vi "SLMLabv1 Test.vi"() -> ()   [LabVIEW 2019]
uses:
  <vilib>/vision/NI_Vision_Development_Module.lvlib
panel:
  in  "N Iterations":i32
  out "N Pixels":i32
  out "SLM Size":i32
  out "startCuda Return":i32
  in  "CUDA":bool
  out "stopCUDA Return":i32
  out "generatePhase Return":i32
  out "Path to Image File":path
  out "Desired Amplitude":sgl[][](array[numeric])
  in  "Update":bool
  out "Path to CUDA DLL":path
  out "Desired Amplitude":T1(plugin-control)
  in  "Stop":bool
  out "Phase SLM":T1(plugin-control)
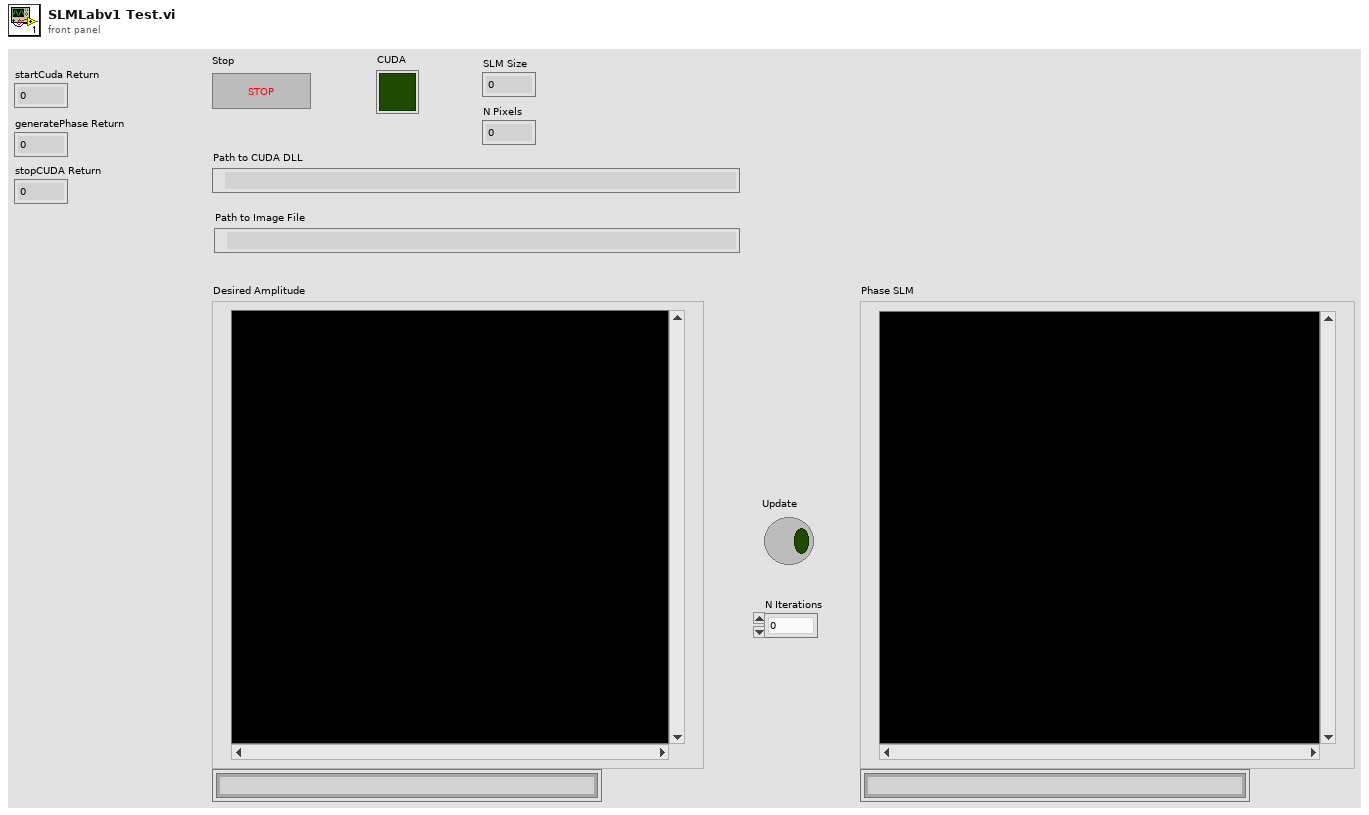
[diagram p1: front panel]
types:
  T1 = typedef "IMAQ Image.ctl" = refnum<image>
  T2 = typedef "Image Type" = u32
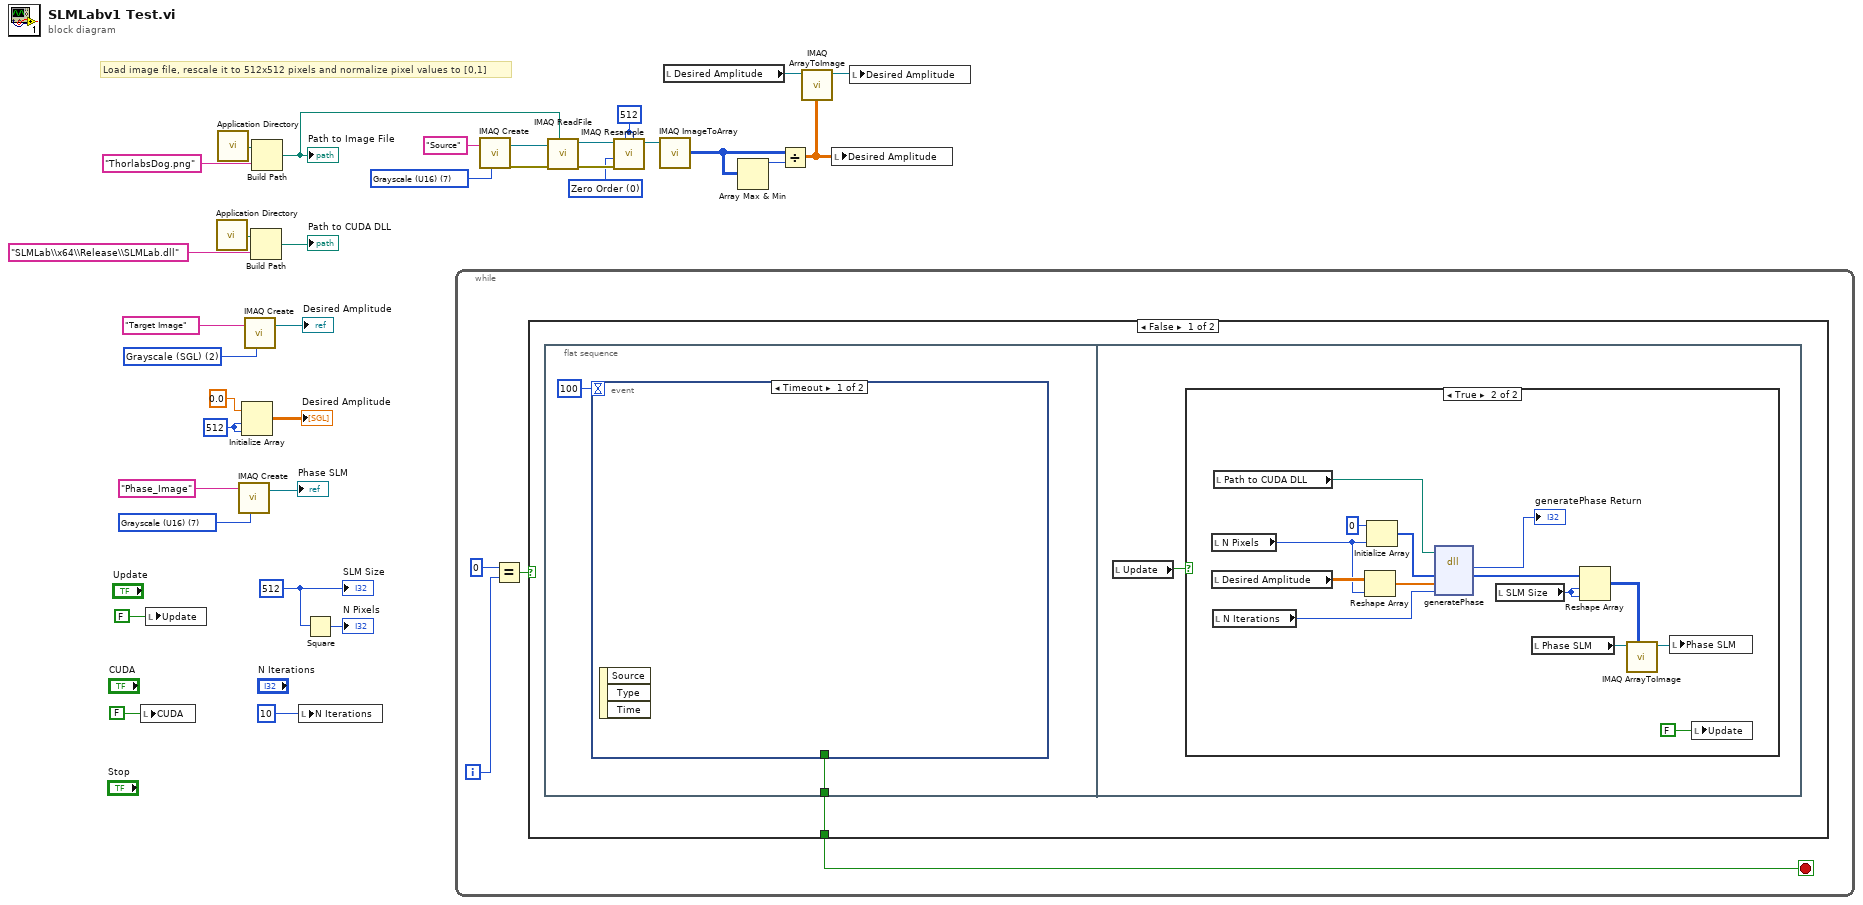
[diagram p0: block diagram]
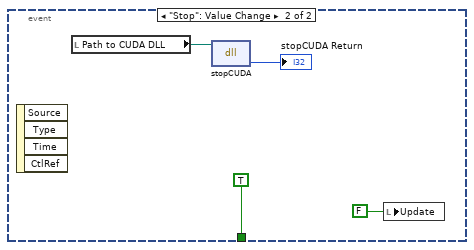
[diagram p2: hidden frame]
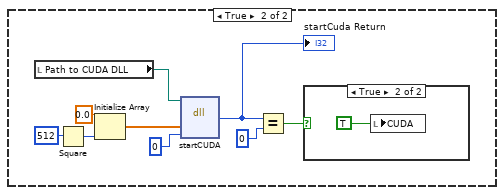
[diagram p4: hidden frame]
diagram:
  w2 = 512
  w15 = T2 7 items=["Grayscale (U8)", "Grayscale (I16)", "Grayscale (SGL)", "Complex (CSG)", "RGB (U32)", "HSL (U32)", "RGB (U64)", "Grayscale (U16)"] ("Image Type")
  w12 = 512
  w11 = u32 0 items=["Zero Order", "Bi-Linear", "Quadratic", "Cubic Spline"] ("Interpolation Type")
  w23 = 512 ("dimension size")
  w29 = T2 2 items=["Grayscale (U8)", "Grayscale (I16)", "Grayscale (SGL)", "Complex (CSG)", "RGB (U32)", "HSL (U32)", "RGB (U64)", "Grayscale (U16)"] ("Image Type")
  w33 = T2 7 items=["Grayscale (U8)", "Grayscale (I16)", "Grayscale (SGL)", "Complex (CSG)", "RGB (U32)", "HSL (U32)", "RGB (U64)", "Grayscale (U16)"] ("Image Type")
  # "Load image file, rescale it to 512x512 pixels and normalize pixel values to [0,1]"
  n1 = local write "CUDA"(FALSE ("Update SLM")) -> ()
  n2 = local write "Update"(FALSE ("Update SLM")) -> ()
  n3 = call <vilib>:"Application Directory.vi"() -> ("Application Directory"=w26:path)
  n4 = call <vilib>:"Application Directory.vi"() -> ("Application Directory"=w7:path)
  n5 = call "IMAQ Create"("Image Name"="Phase_Image", "Image Type"=w33) -> ("New Image"=→"Phase SLM":T1)  [unwired: 3 in, 1 out]
  n6 = Initialize Array(sgl 0.0, w23, w23) -> (→"Desired Amplitude":sgl[][])
  n7 = call "IMAQ Create"("Image Name"="Target Image", "Image Type"=w29) -> ("New Image"=→"Desired Amplitude":T1)  [unwired: 3 in, 1 out]
  n8 = Build Path(base path=w26, name or relative path="SLMLab\\x64\\Release\\SLMLab.dll") -> (appended path=→"Path to CUDA DLL":path)
  n9 = Build Path(base path=w7, name or relative path="ThorlabsDog.png") -> (appended path=w4:path)
  "Path to Image File" <- w4
  n10 = local write "N Iterations"(10) -> ()
  n11 = Square(x=w2) -> (x^2=→"N Pixels":i32)
  n12 = while {
    i -> [w36]
    stop <- w35 stop-if-true
    n13 = Equal?(x=0, y=w36) -> (x = y?=w37:bool)
    n14 = case shown="False" w37 {
      tunnel: [w39 _] -> w35
      frame False {
        n15 = flat-sequence {
          tunnel: [w41] -> w39
          frame #0 {
            n16 = event shown="[0] Timeout" {
              selector: _ -> [_ _]
              dyn-events: _ -> [_ _]
              timeout: 100 -> [_ _]
              tunnel: [_ TRUE] -> w41
              event Timeout {
                n17 = event-data() -> ()  [unwired: 1 in, 3 out]
              }
              event "Stop": Value Change {
                n18 = event-data() -> ()  [unwired: 1 in, 4 out]
                n19 = local read "Path to CUDA DLL"() -> (w43:path)
                n20 = dll-call lib="?" fn="stopCUDA"(path in=w43) -> ("Return Value"=→"stopCUDA Return":i32)  [unwired: 2 in, 2 out]
                n21 = local write "Update"(FALSE ("Update SLM")) -> ()
              }
            }
          }
          frame #1 {
            n22 = local read "Update"() -> (w46:bool)
            n23 = case shown="True" w46 {
              frame False {
              }
              frame True {
                n24 = local read "N Pixels"() -> (w49:i32)
                n25 = local read "Desired Amplitude"() -> (w60:sgl[][])
                n26 = local read "N Iterations"() -> (w47:i32)
                n27 = local read "Path to CUDA DLL"() -> (w51:path)
                n28 = Reshape Array(w60, w49) -> (w59:sgl[])
                n29 = Initialize Array(u16 0 ("element"), w49) -> (w52:u16[])
                n30 = dll-call lib="?" fn="generatePhase"(path in=w51, "h_pSLM_uint16"=w52, "h_dAmplitude"=w59, "n_iterations"=w47) -> ("Return Value"=→"generatePhase Return":i32, "h_pSLM_uint16"=w57:u16[])  [unwired: 4 in, 2 out]
                n31 = local read "SLM Size"() -> (w48:i32)
                n32 = local read "Phase SLM"() -> (w54:T1)
                n33 = Reshape Array(w57, w48, w48) -> (w56:u16[][])
                n34 = call "IMAQ ArrayToImage"("Image Pixels (U16)"=w56, "Image"=w54) -> ("Image Out"=w55:T1)  [unwired: 8 in, 1 out]
                n35 = local write "Phase SLM"(w55) -> ()
                n36 = local write "Update"(FALSE ("Update SLM")) -> ()
              }
            }
          }
        }
      }
      frame True {
        n37 = local read "Path to CUDA DLL"() -> (w64:path)
        n38 = Square(x=512 ("dimension size")) -> (x^2=w67:i32)
        n39 = Initialize Array(sgl 0.0 ("element"), w67) -> (w65:sgl[])
        n40 = dll-call lib="?" fn="startCUDA"(path in=w64, "h_pSLMstart"=w65, "deviceID"=0) -> ("Rückgabetyp"=w63:i32)  [unwired: 4 in, 2 out]
        "startCuda Return" <- w63
        n41 = Equal?(x=w63, y=0) -> (x = y?=w61:bool)
        n42 = case shown="True" w61 {
          frame False {
          }
          frame True {
            n43 = local write "CUDA"(TRUE ("Update SLM")) -> ()
          }
        }
      }
    }
  }
  n44 = call "IMAQ Create"("Image Name"="Source", "Image Type"=w15) -> ("New Image"=w8:T1, "error out"=w9:errorcluster)  [unwired: 3 in]
  n45 = call "IMAQ ReadFile"("File Path"=w4, "error in (no error)"=w9, "Image"=w8) -> ("error out"=w14:errorcluster, "Image Out"=w10:T1)  [unwired: 4 in, 3 out]
  n46 = call "IMAQ Resample"("X Resolution"=w12, "Y Resolution"=w12, "error in (no error)"=w14, "Interpolation Type"=w11, "Image Src"=w10) -> ("Image Dst Out"=w18:T1)  [unwired: 5 in, 1 out]
  n47 = call "IMAQ ImageToArray"("Image"=w18) -> ("Image Pixels (U16)"=w5:u16[][])  [unwired: 3 in, 4 out]
  n48 = local read "Desired Amplitude"() -> (w19:T1)
  n49 = Array Max & Min(array=w5) -> (max value=w16:u16)  [unwired: 3 out]
  n50 = Divide(x=w5, y=w16) -> (x/y=w17:dbl[][])
  n51 = call "IMAQ ArrayToImage"("Image Pixels (Float)"=w17, "Image"=w19) -> ("Image Out"=w20:T1)  [unwired: 8 in, 1 out]
  n52 = local write "Desired Amplitude"(w17) -> ()
  n53 = local write "Desired Amplitude"(w20) -> ()
  "SLM Size" <- w2
